vi "StateLimeLight.vi"(0 "Master State In":T1(ring)) -> ()   [LabVIEW 2023]
doc: "This VI manages the LimeLight pipelines and LimeLight targeting LED mode."
uses:
  GlobalMiscellaneous.vi
  GlobalDriverStationData.vi
  GlobalPoseAndTargeting.vi
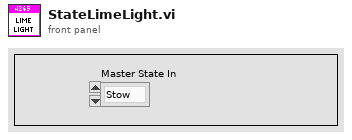
[diagram p1: front panel]
types:
  T1 = enum16{"Stow", "Speaker", "Amp", "Climbing", "Trap"}
  T2 = enum16{"Side-by-Side", "PiP Main", "PiP Secondary"}
  T3 = enum16{"Boot Up", "Camera Override", "AprilTags", "Gamepiece Tracking"}
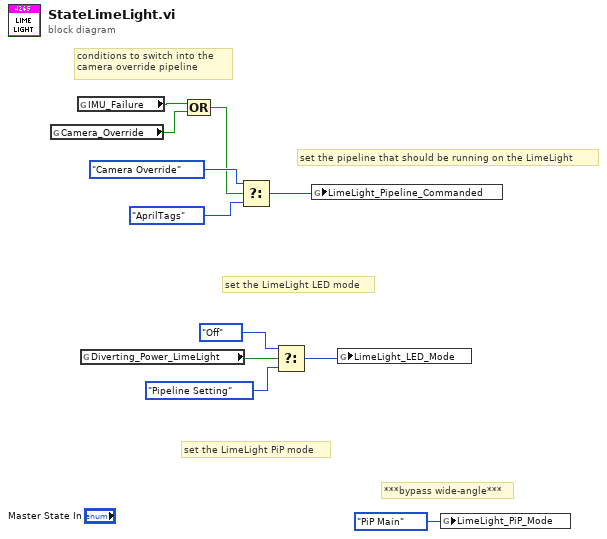
[diagram p0: block diagram]
diagram:
  # "***bypass wide-angle***"
  # "set the LimeLight PiP mode"
  # "set the LimeLight LED mode"
  # "conditions to switch into the \ncamera override pipeline"
  # "set the pipeline that should be running on the LimeLight"
  n1 = global read "GlobalDriverStationData.vi" "Camera_Override"() -> (w10:bool)
  n2 = global read "GlobalPoseAndTargeting.vi" "IMU_Failure"() -> (w11:bool)
  n3 = global read "GlobalMiscellaneous.vi" "Diverting_Power_LimeLight"() -> (w5:bool)
  n4 = Compound Arithmetic op=OR(w11, w10) -> (w8:bool)
  n5 = Select(t=T3."Camera Override", s=w8, f=T3."AprilTags") -> (s? t:f=w4:T3)
  n6 = Select(t=enum16{"Pipeline Setting", "Off", "Blink", "On"}."Off", s=w5, f=enum16{"Pipeline Setting", "Off", "Blink", "On"}."Pipeline Setting") -> (s? t:f=w3:enum16{"Pipeline Setting", "Off", "Blink", "On"})
  n7 = global write "GlobalMiscellaneous.vi" "LimeLight_Pipeline_Commanded"(w4) -> ()
  n8 = global write "GlobalMiscellaneous.vi" "LimeLight_LED_Mode"(w3) -> ()
  n9 = global write "GlobalMiscellaneous.vi" "LimeLight_PiP_Mode"(T2."PiP Main" ("LimeLight_PiP_Mode")) -> ()
